vi "DDGImage.VI"() -> ()   [LabVIEW 2015]
panel:
  out "Intensity Graph":i32[][](graph)
  out "Calculated Kinetic Cycle Time":sgl format="%.2f"
  in  "Frequency (Hz):":dbl format="%.2f"
  in  "Integrate on chip":bool
  in  "Intelligate":bool
  in  "Fast insertion delay":bool
  in  "Gate step (nsecs)":i32 step=25
  in  "Pulse Width (nsecs)":i32=1000
  in  "Delay (nsecs)":i32 step=25
  in  "Output A Delay (nsecs)":i32 min=0 step=16
  in  "Gain (0-255)":i32 min=0 max=255
  in  "Kinetic Cycle Time":sgl format="%.2f"
  in  "Shut Down":bool
  in  "Start Acquisition":bool
  out "Return  from Get Acquired Data":u32
  out "Detector X Pixels":i32
  out "Return from GetStatus":u32
  out "Return from Start Acquisition":u32
  in  "Number of Kinetics":i32=5
  out "Return from CheckTimings Exposure":u32
  out "Calculated Exposure Value":sgl format="%.2f"
  in  "Exposure Time (secs)":sgl=0.05 format="%.2f"
  out "Return from Initialize":u32
  in  "Trigger":u32(ring) items=["Internal", "External"]
  # "Acquisition Mode: Kinetics\nReadout Mode: Full Image.  Only showing one image of data."
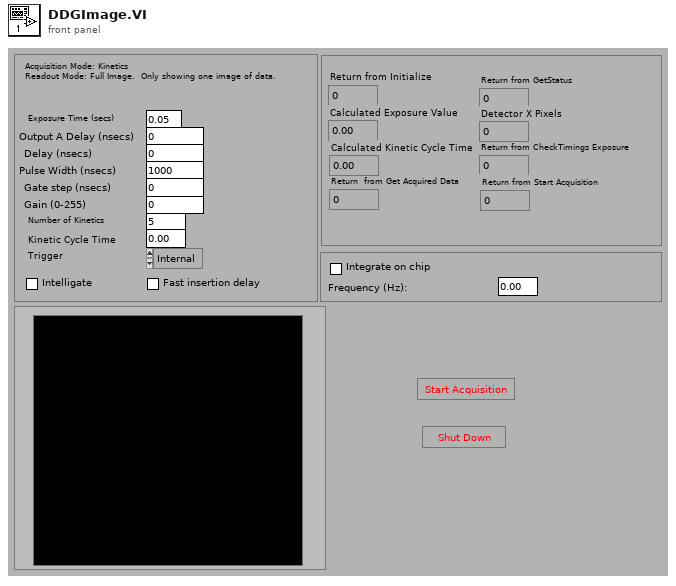
[diagram p1: front panel]
types:
  T1 = typedef "Error Code Enum typedef.ctl" = enum32{"N/A (0)", "DRV_ERROR_CODES", "DRV_SUCCESS", "DRV_VXDNOTINSTALLED", "DRV_ERROR_SCAN", "DRV_ERROR_CHECK_SUM", "DRV_ERROR_FILELOAD", "DRV_UNKNOWN_FUNC", "DRV_ERROR_VXD_INIT", "DRV_ERROR_ADDRESS", "DRV_ERROR_PAGELOCK", "DRV_ERROR_PAGEUNLOCK", "DRV_ERROR_BOARDTEST", "DRV_ERROR_ACK", "DRV_ERROR_UP_FIFO", "DRV_ERROR_PATTERN", "N/A (16)", "DRV_ACQUISITION_ERRORS", "DRV_ACQ_BUFFER", "DRV_ACQ_DOWNFIFO_FULL", "DRV_PROC_UNKONWN_INSTRUCTION", "DRV_ILLEGAL_OP_CODE", "DRV_KINETIC_TIME_NOT_MET", "DRV_ACCUM_TIME_NOT_MET", "DRV_NO_NEW_DATA", "N/A (25)", "DRV_SPOOLERROR", "N/A (27)", "N/A (28)", "N/A (29)", "N/A (30)", "N/A (31)", "N/A (32)", "DRV_TEMPERATURE_CODES", "DRV_TEMPERATURE_OFF", "DRV_TEMPERATURE_NOT_STABILIZED", "DRV_TEMPERATURE_STABILIZED", "DRV_TEMPERATURE_NOT_REACHED", "DRV_TEMPERATURE_OUT_RANGE", "DRV_TEMPERATURE_NOT_SUPPORTED", "DRV_TEMPERATURE_DRIFT", "N/A (41)", "N/A (42)", "N/A (43)", "N/A (44)", "N/A (45)", "N/A (46)", "N/A (47)", "N/A (48)", "DRV_GENERAL_ERRORS", "DRV_INVALID_AUX", "DRV_COF_NOTLOADED", "DRV_FPGAPROG", "DRV_FLEXERROR", "DRV_GPIBERROR", "N/A (55)", "N/A (56)", "N/A (57)", "N/A (58)", "N/A (59)", "N/A (60)", "N/A (61)", "N/A (62)", "N/A (63)", "DRV_DATATYPE", "DRV_DRIVER_ERRORS", "DRV_P1INVALID", "DRV_P2INVALID", "DRV_P3INVALID", "DRV_P4INVALID", "DRV_INIERROR", "DRV_COFERROR", "DRV_ACQUIRING", "DRV_IDLE", "DRV_TEMPCYCLE", "DRV_NOT_INITIALIZED", "DRV_P5INVALID", "DRV_P6INVALID", "DRV_INVALID_MODE", "DRV_INVALID_FILTER", "DRV_I2CERRORS", "DRV_I2CDEVNOTFOUND", "DRV_I2CTIMEOUT", "DRV_P7INVALID", "N/A (84)", "N/A (85)", "N/A (86)", "N/A (87)", "N/A (88)", "N/A (89)", "DRV_IOCERROR", "DRV_VRMVERSIONERROR"}
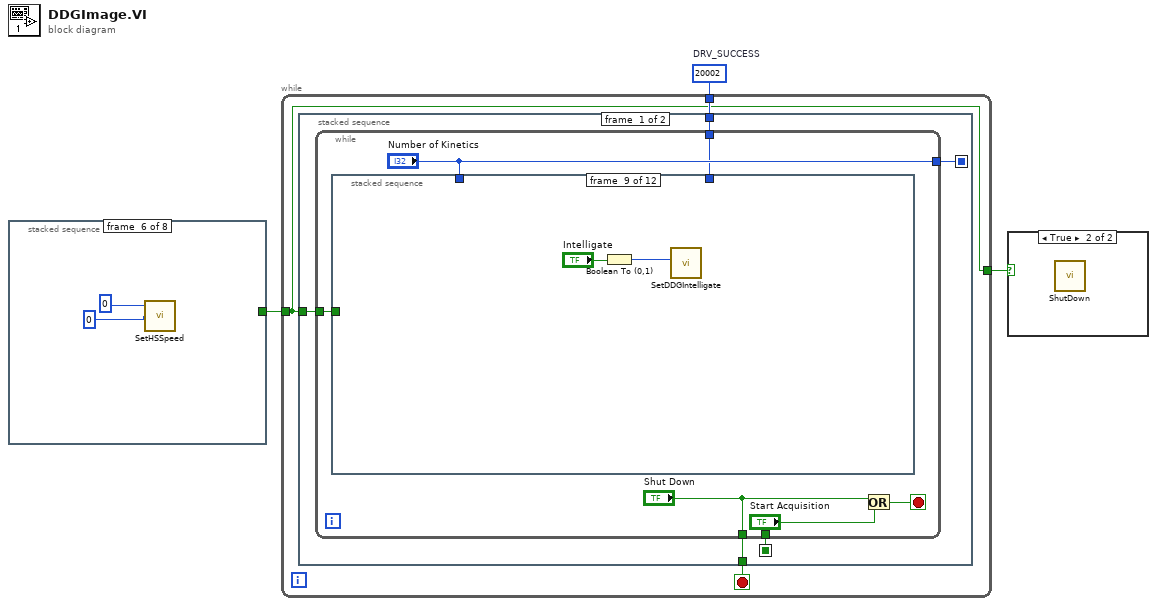
[diagram p0: block diagram]
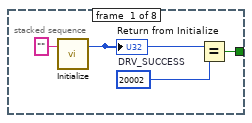
[diagram p2: hidden frame]
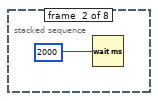
[diagram p3: hidden frame]
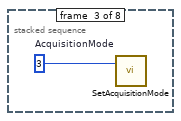
[diagram p4: hidden frame]
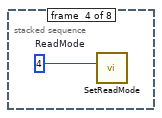
[diagram p5: hidden frame]
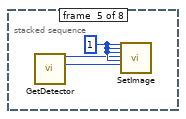
[diagram p6: hidden frame]
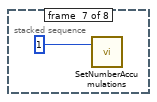
[diagram p7: hidden frame]
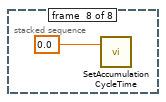
[diagram p8: hidden frame]
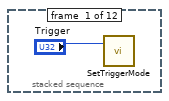
[diagram p10: hidden frame]
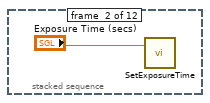
[diagram p11: hidden frame]
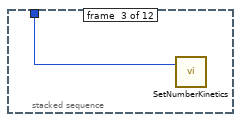
[diagram p12: hidden frame]
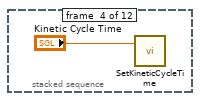
[diagram p13: hidden frame]
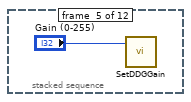
[diagram p14: hidden frame]
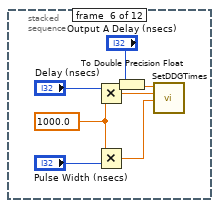
[diagram p15: hidden frame]
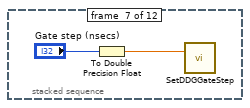
[diagram p16: hidden frame]
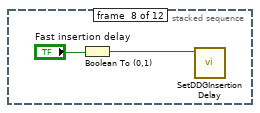
[diagram p17: hidden frame]
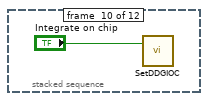
[diagram p18: hidden frame]
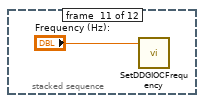
[diagram p19: hidden frame]
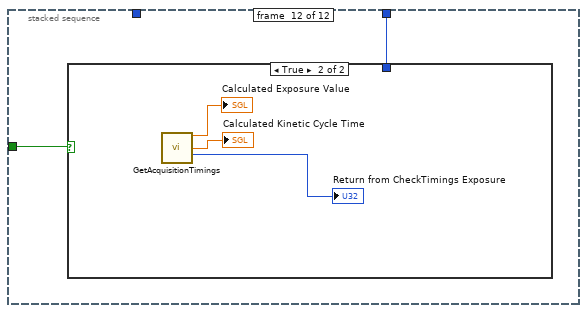
[diagram p20: hidden frame]
diagram:
  w1 = 20002  # DRV_SUCCESS
  n1 = stacked-sequence {
    tunnel: [w4 _ _ _ _ _ _ _] -> w2
    frame #0 {
      w5 = 20002  # DRV_SUCCESS
      n2 = call "Initialize.vi"("directory (\"\")"="" ("directory (\"\")")) -> ("DLL error code"=w6:u32)  [unwired: 1 in, 1 out]
      "Return from Initialize" <- w6
      n3 = Equal?(x=w6, y=w5) -> (x = y?=w4:bool)
    }
    frame #1 {
      n4 = Wait (ms)(milliseconds to wait=u32 2000) -> ()  [unwired: 1 out]
    }
    frame #2 {
      w9 = u16 3  # AcquisitionMode
      n5 = call "SetAcquisitionMode.vi"("mode"=w9) -> ()  [unwired: 1 in, 2 out]
    }
    frame #3 {
      w10 = u16 4  # ReadMode
      n6 = call "SetReadMode.vi"("mode"=w10) -> ()  [unwired: 1 in, 2 out]
    }
    frame #4 {
      w13 = 1
      n7 = call "GetDetector.vi"() -> ("ypixels"=w11:i32, "xpixels"=w12:i32)  [unwired: 4 in, 2 out]
      n8 = call "SetImage.vi"("hbin"=w13, "vbin"=w13, "hstart"=w13, "hend"=w12, "vstart"=w13, "vend"=w11) -> ()  [unwired: 20 in, 2 out]
    }
    frame #5 {
      n9 = call "SetHSSpeed.vi"("index"=0, "type"=0) -> ()  [unwired: 2 in, 2 out]
    }
    frame #6 {
      n10 = call "SetNumberAccumulations.vi"("number"=1) -> ()  [unwired: 1 in, 2 out]
    }
    frame #7 {
      n11 = call "SetAccumulationCycleTime.vi"("time"=sgl 0.0) -> ()  [unwired: 1 in, 2 out]
    }
  }
  n12 = while {
    tunnel: [w18] -> w3
    tunnel: w2 -> [w18]
    tunnel: w1 -> [w19]
    stop <- w20 stop-if-true
    n13 = stacked-sequence {
      seq-local: [w24 _] -> [_ w59]
      seq-local: [w21 _] -> [_ w57]
      tunnel: [w25 _] -> w20
      tunnel: w18 -> [w23 _]
      tunnel: w19 -> [w22 w58]
      frame #0 {
        n14 = while {
          tunnel: ["Shut Down"] -> w25
          tunnel: ["Number of Kinetics"] -> w24
          tunnel: w23 -> [w28]
          tunnel: w22 -> [w27]
          tunnel: ["Start Acquisition"] -> w21
          stop <- w31 stop-if-true
          n15 = stacked-sequence {
            tunnel: "Number of Kinetics" -> [_ _ w34 _ _ _ _ _ _ _ _ _]
            tunnel: w28 -> [_ _ _ _ _ _ _ _ _ _ _ w53]
            tunnel: w27 -> [_ _ _ _ _ _ _ _ _ _ _ w52]
            frame #0 {
              n16 = call "SetTriggerMode.vi"("mode"="Trigger") -> ()  [unwired: 1 in, 2 out]
            }
            frame #1 {
              n17 = call "SetExposureTime.vi"("time"="Exposure Time (secs)") -> ()  [unwired: 1 in, 2 out]
            }
            frame #2 {
              n18 = call "SetNumberKinetics.vi"("number"=w34) -> ()  [unwired: 1 in, 2 out]
            }
            frame #3 {
              n19 = call "SetKineticCycleTime.vi"("time"="Kinetic Cycle Time") -> ()  [unwired: 1 in, 2 out]
            }
            frame #4 {
              n20 = call "SetDDGGain.vi"("gain"="Gain (0-255)") -> ()  [unwired: 1 in, 2 out]
            }
            frame #5 {
              w39 = 1000.0
              n21 = Multiply(x="Delay (nsecs)", y=w39) -> (x*y=w37:dbl)
              n22 = Multiply(x=w39, y="Pulse Width (nsecs)") -> (x*y=w38:dbl)
              n23 = To Double Precision Float(number="Output A Delay (nsecs)") -> (double precision float=w42:dbl)
              n24 = call "SetDDGTimes.vi"("T2"=w38, "T1"=w37, "T0"=w42) -> ()  [unwired: 3 in, 2 out]
            }
            frame #6 {
              n25 = To Double Precision Float(number="Gate step (nsecs)") -> (double precision float=w44:dbl)
              n26 = call "SetDDGGateStep.vi"("step"=w44) -> ()  [unwired: 1 in, 2 out]
            }
            frame #7 {
              n27 = Boolean To (0,1)(Boolean="Fast insertion delay") -> (0, 1=w46:i16)
              n28 = call "SetDDGInsertionDelay.vi"("State"=w46) -> ()  [unwired: 9 in, 2 out]
            }
            frame #8 {
              n29 = Boolean To (0,1)(Boolean="Intelligate") -> (0, 1=w48:i16)
              n30 = call "SetDDGIntelligate.vi"("State"=w48) -> ()  [unwired: 9 in, 2 out]
            }
            frame #9 {
              n31 = call "SetDDGIOC.vi"("integrate"="Integrate on chip") -> ()  [unwired: 1 in, 2 out]
            }
            frame #10 {
              n32 = call "SetDDGIOCFrequency.vi"("frequency"="Frequency (Hz):") -> ()  [unwired: 1 in, 2 out]
            }
            frame #11 {
              n33 = case shown="True" w53 {
                tunnel: w52 -> [_ _]
                frame False {
                }
                frame True {
                  n34 = call "GetAcquisitionTimings.vi"() -> ("exposure"=→"Calculated Exposure Value":sgl, "kinetic"=→"Calculated Kinetic Cycle Time":sgl, "DLL error code"=→"Return from CheckTimings Exposure":u32)  [unwired: 11 in, 2 out]
                }
              }
            }
          }
          n35 = Or(x="Shut Down", y="Start Acquisition") -> (x .or. y?=w31:bool)
        }
      }
      frame #1 {
        n36 = stacked-sequence {
          seq-local: [w61 _ _] -> [_ w67 _]
          tunnel: w58 -> [w62 _ _]
          tunnel: w57 -> [w60 _ _]
          tunnel: w59 -> [_ _ w80]
          frame #0 {
            n37 = case shown="True" w60 {
              tunnel: [FALSE w66] -> w61
              tunnel: w62 -> [_ w64]
              frame False {
              }
              frame True {
                n38 = call "StartAcquisition.vi"() -> ("DLL error code"=w65:u32)  [unwired: 2 in, 1 out]
                "Return from Start Acquisition" <- w65
                n39 = Equal?(x=w64, y=w65) -> (x = y?=w66:bool)
              }
            }
          }
          frame #1 {
            n40 = case shown="True" w67 {
              frame False {
              }
              frame True {
                n41 = while {
                  stop <- w70 continue-if-true
                  w69 = u16 72  # DRV ACQUIRING
                  n42 = Wait Until Next ms Multiple(millisecond multiple=u32 50) -> ()  [unwired: 1 out]
                  n43 = call "GetStatus.vi"() -> ("status"=w68:T1)  [unwired: 3 in, 2 out]
                  "Return from GetStatus" <- w68
                  n44 = Equal?(x=w68, y=w69) -> (x = y?=w70:bool)
                }
              }
            }
          }
          frame #2 {
            n45 = call "GetDetector.vi"() -> ("ypixels"=w73:i32, "xpixels"=w74:i32)  [unwired: 4 in, 2 out]
            "Detector X Pixels" <- w74
            n46 = Multiply(x=w74, y=w73) -> (x*y=w76:i32)
            n47 = Multiply(x=w80, y=w76) -> (x*y=w79:i32)
            n48 = call "GetAcquiredData.vi"("size"=w79) -> ("DLL error code"=→"Return  from Get Acquired Data":u32, "array"=w78:i32[])  [unwired: 2 in, 1 out]
            n49 = Array Subset(array=w78, index=0, length=w76) -> (w75:i32[])
            n50 = Reshape Array(w75, w74, w73) -> (→"Intensity Graph":i32[][])
          }
        }
      }
    }
  }
  n51 = case shown="True" w3 {
    frame False {
    }
    frame True {
      n52 = call "ShutDown.vi"() -> ()  [unwired: 2 in, 2 out]
    }
  }
